vi "全局 1.vi"() -> ()   [LabVIEW 2018]
panel:
  in  "旋转":dbl
  in  "升降":dbl
  in  "抱爪2":dbl
  in  "抱爪1":dbl
  in  "换向阀 2":dbl
  in  "灯4":dbl
  in  "灯56":dbl
  in  "灯34":dbl
  in  "灯12":dbl
  in  "换向阀":dbl
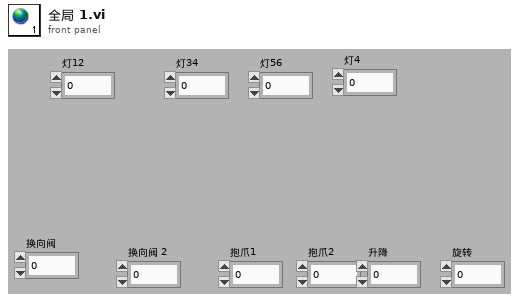
[diagram p1: front panel]
diagram:
